vi "hdt_aux_averageChannels.vi"(11 "enableOutput":bool) -> ()   [LabVIEW 2016]
uses:
  <vilib>/rvi/Emulation/niFpgaEmulationIsFPGAContextNoSignature.vi
  <vilib>/rvi/Emulation/niFpgaSctlEmulationGetInTimedLoop.vi
  <vilib>/rvi/errors/niFpgaSetErrorForExecOnDevCompSimple.vi
  <vilib>/rvi/eio/common/nirviEmuReportErrorAndStop.vi
  <vilib>/rvi/DataTransferAndStorage/Container/Common/niFpgaContainerGetUniqueNameForEmu.vi
  <vilib>/rvi/FIFO/Fifo_Resource/nirvififoEmulationSetSize.vi
  <vilib>/rvi/FIFO/Fifo_Resource/nirviFifoEmulationQueueMgr.vi
  <instcachedir>/0/nirviFifoEmulationQueueMgr_E5CAEC123FF24DC58D834DCA3CDAA9B5.lvgen/nirviFifoEmulationQueueMgr_E5CAEC123FF24DC58D834DCA3CDAA9B5_010.vi
  <vilib>/Utility/error.llb/Clear Errors.vi
  <vilib>/rvi/FIFO/Fifo_Resource/nirvififoEmulationCreateLock.vi
  <vilib>/rvi/Emulation/niFpgaProcessEmulError.vi
  <vilib>/rvi/FIFO/Fifo_Resource/nirvififoEmulationObtainLock.vi
  <vilib>/rvi/FIFO/Fifo_Resource/nirvififoEmulationReleaseLock.vi
  <vilib>/rvi/occurrence/nirviWaitOnOccurrenceBase.vi
  <vilib>/rvi/errors/nirviReportUnexpectedCaseInternalError.vi
  <vilib>/rvi/errors/nirviReportUnexpectedCaseInternalError (U32).vi
  <instcachedir>/0/nirviFifoEmulationQueueMgr_E5CAEC123FF24DC58D834DCA3CDAA9B5.lvgen/nirviFifoEmulationQueueMgr_E5CAEC123FF24DC58D834DCA3CDAA9B5_009.vi
  <vilib>/rvi/FIFO/Fifo_Resource/nirvififoEmulationDetermineInputValidOut.vi
  <vilib>/rvi/DataTransferAndStorage/Container/XNode/niFpgaContainer.xnode
  <vilib>/rvi/FIFO/Fifo_Resource/nirvififoEmulationRead.vi
  <vilib>/rvi/FXPMathLib/FxpInterpret/XNode/nifxpmath_Interpret.xnode
  <vilib>/rvi/FIFO/Fifo_Resource/nirvififoEmulationWrite.vi
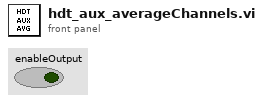
[diagram p1: front panel]
types:
  T1 = cluster{"Element[0]":fxp<+/-,22,1>, "Element[1]":fxp<+/-,22,1>, "Element[2]":fxp<+/-,22,1>, "Element[3]":fxp<+/-,22,1>, "Element[4]":fxp<+/-,22,1>, "Element[5]":fxp<+/-,22,1>, "Element[6]":fxp<+/-,22,1>, "Element[7]":fxp<+/-,22,1>}
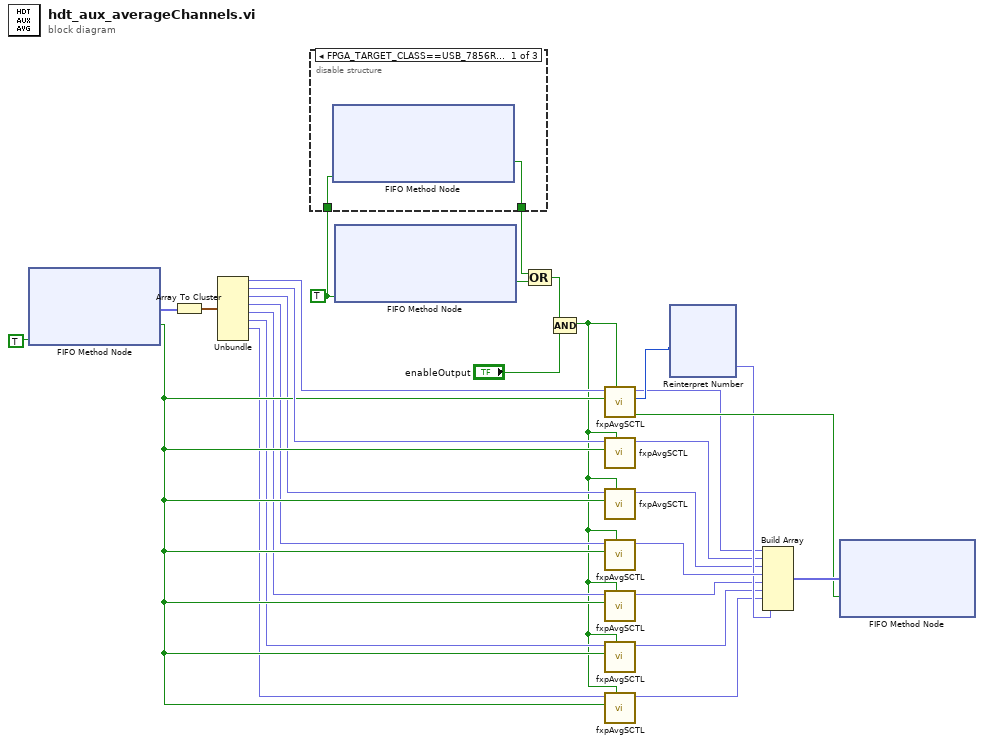
[diagram p0: block diagram]
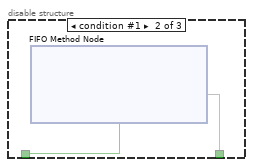
[diagram p2: hidden frame]
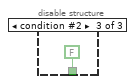
[diagram p3: hidden frame]
diagram:
  w2 = TRUE ("Ready for Output")
  n1 = xnode ("FIFO Method Node")("Ready for Output"=TRUE) -> ("Element"=w17:fxp<+/-,22,1>[], "Output Valid"=w25:bool)  [unwired: 1 in, 1 out]
  n2 = Array To Cluster(array=w17) -> (cluster=w18:T1)
  n3 = Unbundle(w18) -> ("Element[0]"=w19:fxp<+/-,22,1>, "Element[1]"=w26:fxp<+/-,22,1>, "Element[2]"=w20:fxp<+/-,22,1>, "Element[3]"=w21:fxp<+/-,22,1>, "Element[4]"=w22:fxp<+/-,22,1>, "Element[5]"=w23:fxp<+/-,22,1>, "Element[6]"=w24:fxp<+/-,22,1>)  [unwired: 1 out]
  n4 = disable-structure shown="FPGA_TARGET_CLASS==USB_7856R_OEM||FPGA_TARGET_CLASS==USB_7856R" {
    disable-tunnel: w2 -> [w30 w32 _]
    disable-tunnel: [w29 w31 FALSE ("Output Valid")] -> w1
    frame condition #0 (active) {
      n5 = xnode ("FIFO Method Node")("Ready for Output"=w30) -> ("Output Valid"=w29:bool)  [unwired: 1 in, 2 out]
    }
    frame condition #1 {
      n6 = xnode ("FIFO Method Node")("Ready for Output"=w32) -> ("Output Valid"=w31)  [unwired: 1 in, 2 out]
    }
    frame condition #2 {
    }
  }
  n7 = xnode ("FIFO Method Node")("Ready for Output"=w2) -> ("Output Valid"=w5:bool)  [unwired: 1 in, 2 out]
  n8 = Compound Arithmetic op=OR(w1, w5) -> (w3:bool)
  n9 = Compound Arithmetic op=AND(w3, "enableOutput") -> (w6:bool)
  n10 = call "fxpAvgSCTL.vi"("reset"=w6, "inputValid"=w25, "input"=w19) -> ("outputValid"=w27:bool, "noAvg"=w13:u16, "average"=w7:fxp<+/-,22,1>)  [unwired: 5 in, 1 out]
  n11 = call "fxpAvgSCTL.vi"("reset"=w6, "inputValid"=w25, "input"=w26) -> ("average"=w8:fxp<+/-,22,1>)  [unwired: 5 in, 3 out]
  n12 = call "fxpAvgSCTL.vi"("reset"=w6, "inputValid"=w25, "input"=w20) -> ("average"=w9:fxp<+/-,22,1>)  [unwired: 5 in, 3 out]
  n13 = call "fxpAvgSCTL.vi"("reset"=w6, "inputValid"=w25, "input"=w21) -> ("average"=w15:fxp<+/-,22,1>)  [unwired: 5 in, 3 out]
  n14 = call "fxpAvgSCTL.vi"("reset"=w6, "inputValid"=w25, "input"=w22) -> ("average"=w10:fxp<+/-,22,1>)  [unwired: 5 in, 3 out]
  n15 = call "fxpAvgSCTL.vi"("reset"=w6, "inputValid"=w25, "input"=w23) -> ("average"=w11:fxp<+/-,22,1>)  [unwired: 5 in, 3 out]
  n16 = call "fxpAvgSCTL.vi"("reset"=w6, "inputValid"=w25, "input"=w24) -> ("average"=w12:fxp<+/-,22,1>)  [unwired: 5 in, 3 out]
  n17 = xnode "Reinterpret Number"("x"=w13) -> ("y"=w14:fxp<+,16,1>)
  n18 = Build Array(w7, w8, w9, w15, w10, w11, w12, w14) -> (w28:fxp<+/-,23,2>[])
  n19 = xnode ("FIFO Method Node")("Element"=w28, "Input Valid"=w27) -> ()  [unwired: 1 in, 2 out]
